vi "Read Level.vi"(11 "Dependency in":refnum<class "Dependency.lvclass">) -> (2 "Level":string, 3 "Dependency out":refnum<class "Dependency.lvclass">)   [LabVIEW 2021, in "smo.lvlib" / "Dependency.lvclass"]
uses:
  Dependency.lvclass
  Dependency.lvclass/Dependency.ctl
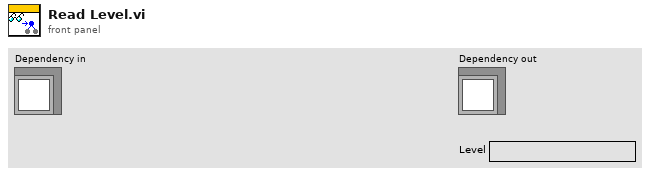
[diagram p1: front panel]
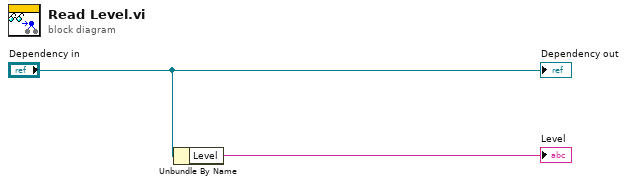
[diagram p0: block diagram]
diagram:
  n1 = Unbundle By Name("Dependency in") -> ("Level"=→"Level":string)
  "Dependency out" <- "Dependency in"
